vi "Spline Interpolant.vi"(2 "final boundary":dbl=1e+30 format="%0.2e", 3 "initial boundary":dbl=1e+30 format="%0.2e", 4 "X":dbl[](array[numeric]) format="%0.2f", 5 "Y":dbl[](array[numeric]) format="%0.2f") -> (0 "error":i32, 1 "Interpolant":dbl[](array[numeric]) format="%0.2f")   [LabVIEW 2020, in "NI_AALPro.lvlib"]
doc: "Returns an array <B>Interpolant</B> of length n, which contains the second derivatives of the spline interpolating function g(x) at the tabulated points x[i], where i = 0, 1, ..., n-1."
uses:
  NI_AALPro.lvlib
  <resource>/lvanlys.dll
panel:
  # "Spline Interpolant"
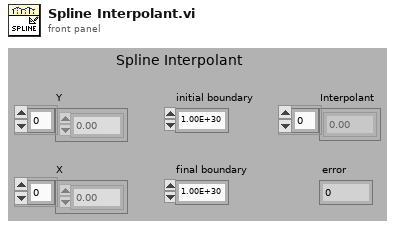
[diagram p1: front panel]
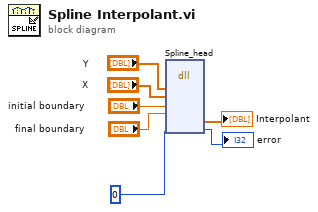
[diagram p0: block diagram]
diagram:
  n1 = dll-call lib="C:/Program Files (x86)/National Instruments/LabVIEW 2020/resource/lvanlys.*" fn="Spline_head"("Y"="Y", "X"="X", "initial boundary"="initial boundary", "final boundary"="final boundary", "output param"=0) -> ("Interpolant"=→"Interpolant":dbl[], "output param"=→"error":i32)  [unwired: 9 in, 2 out]
